vi "Destroy Session.vi"(8 "error in (no error)":errorcluster, 11 "http-client in":refnum<class "http-client.lvclass">) -> (0 "error out":errorcluster)   [LabVIEW 2020, in "http.lvlib" / "http-client.lvclass"]
uses:
  http-client.lvclass
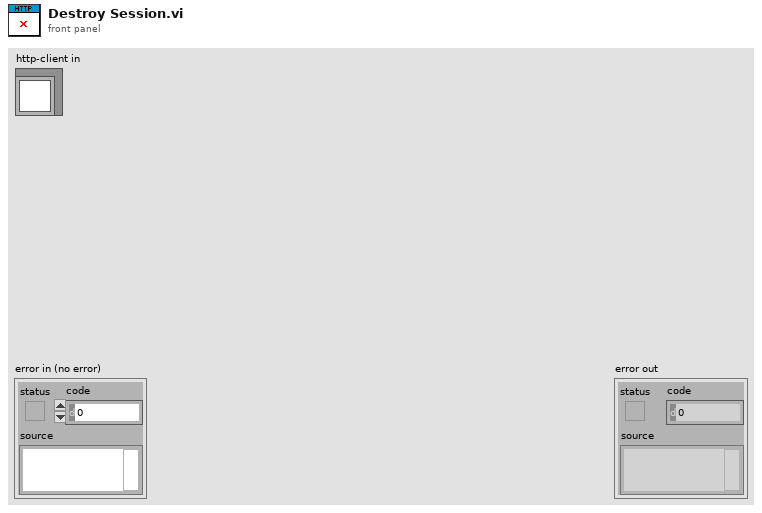
[diagram p1: front panel]
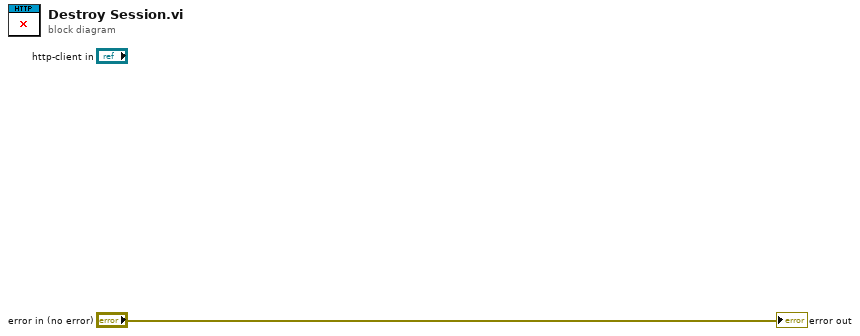
[diagram p0: block diagram]
diagram:
  "error out" <- "error in (no error)"
